vi "战舰胜利界面.vi"() -> ()   [LabVIEW 2018]
panel:
  out "失败界面":picture
  out "胜利界面":picture
  out "敌机是否入侵":bool
  out "得分":dbl
  out "战舰爆炸":picture
  out "血量":dbl
  out "战舰血量":T1 scale=0.0..100.0
  out "敌机爆炸":picture
  in  "敌机数量":dbl
  in  "敌机速度":dbl
  out "敌机":picture
  out "按键":dbl
  out "战舰":T2
  out "激光武器1":T3
  out "激光武器 2":T3
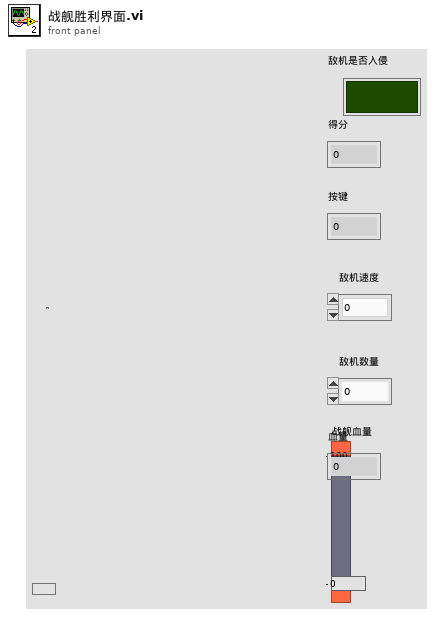
[diagram p1: front panel]
types:
  T1 = typedef "战列巡洋舰_血条.ctl" = dbl
  T2 = typedef "战列巡洋舰.ctl" = picture
  T3 = typedef "战列巡洋舰_激光武器.ctl" = picture
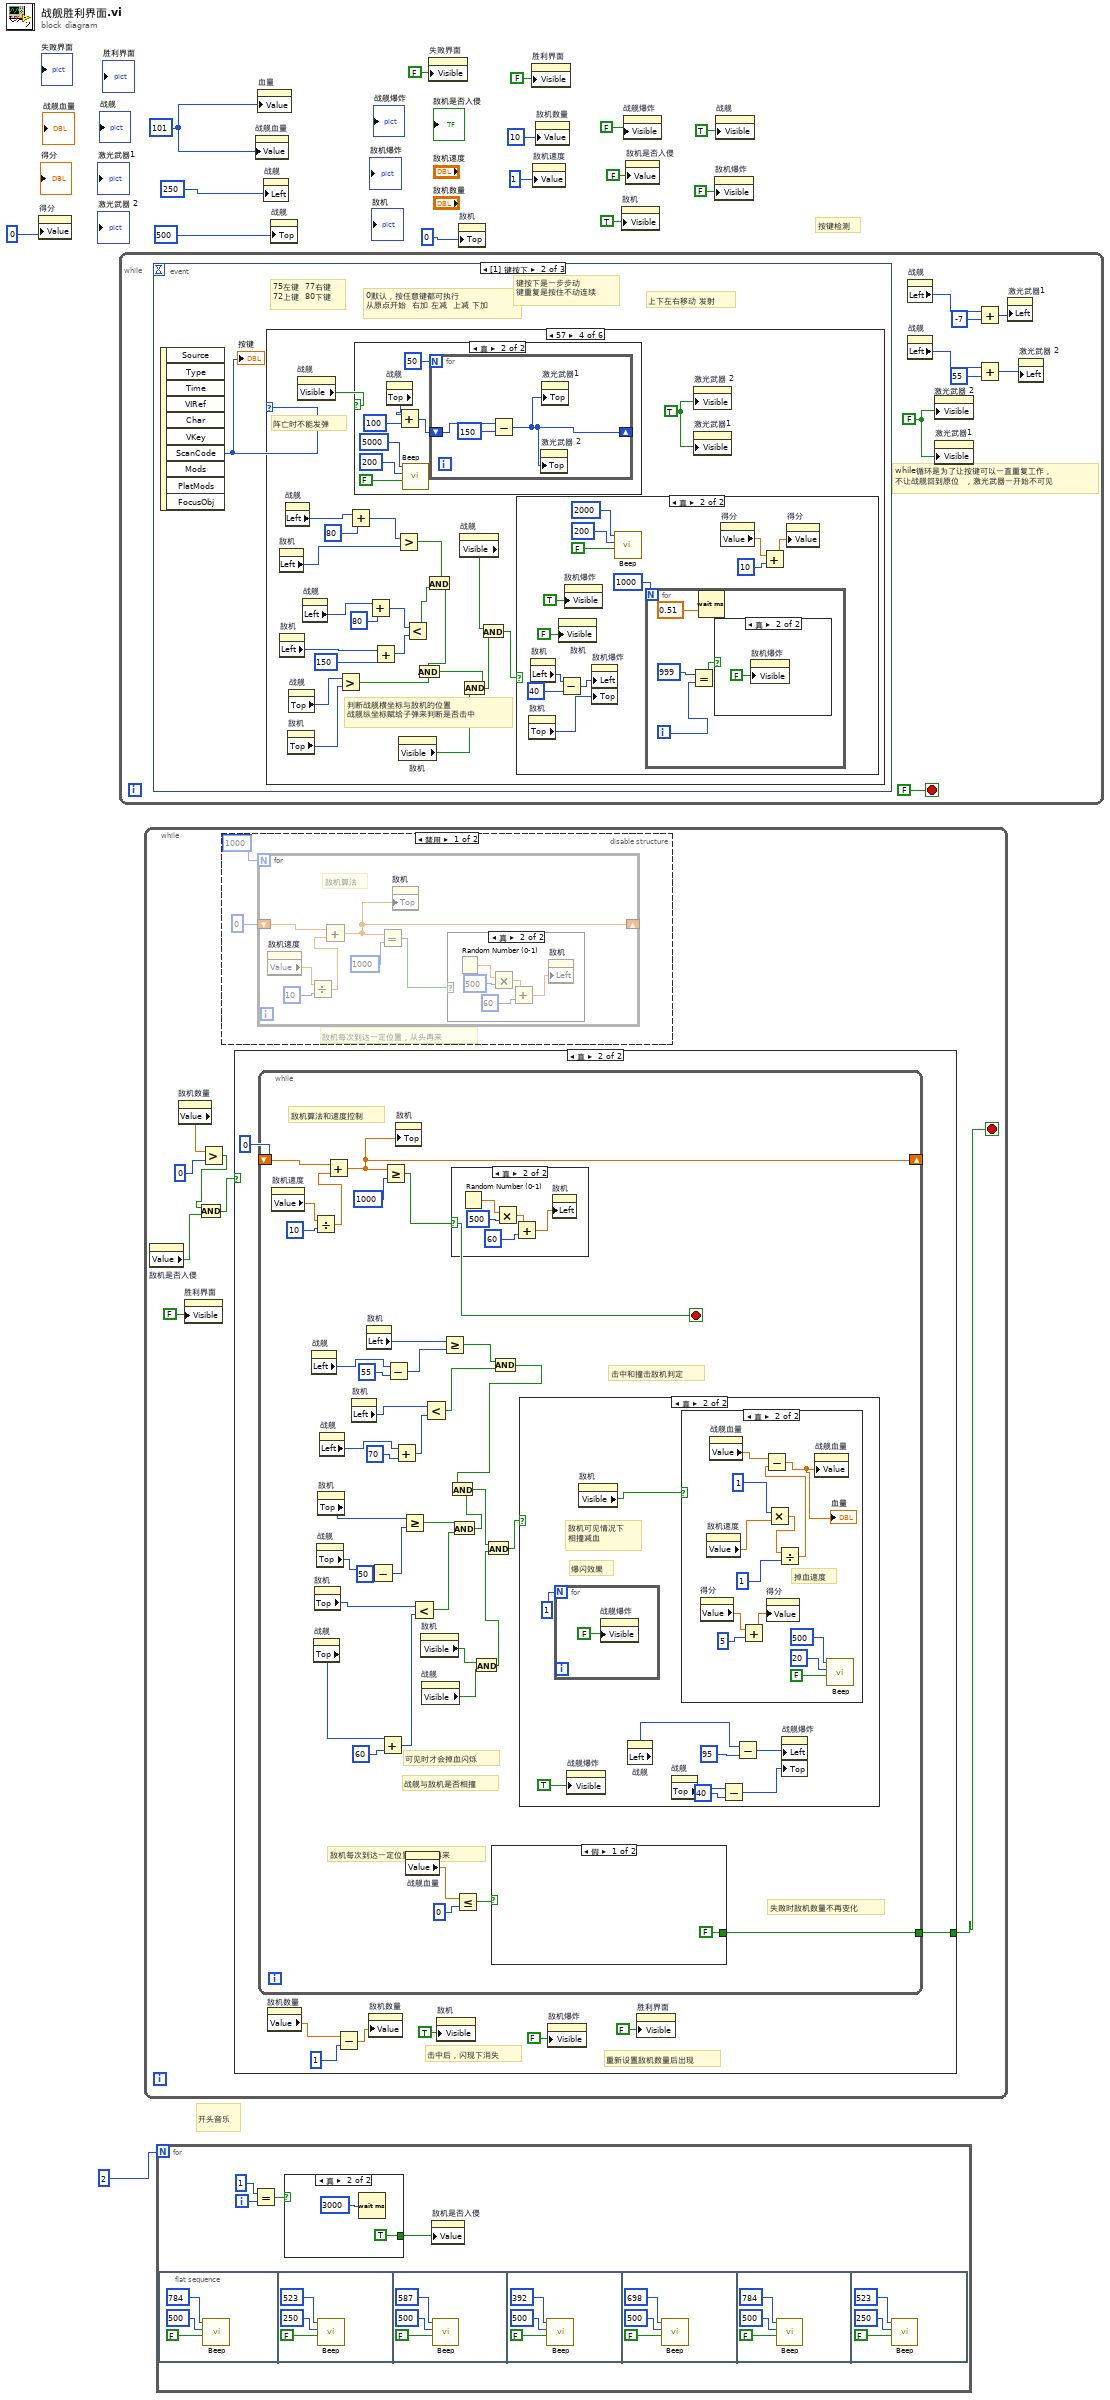
[diagram p0: block diagram]
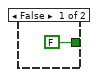
[diagram p2: hidden frame]
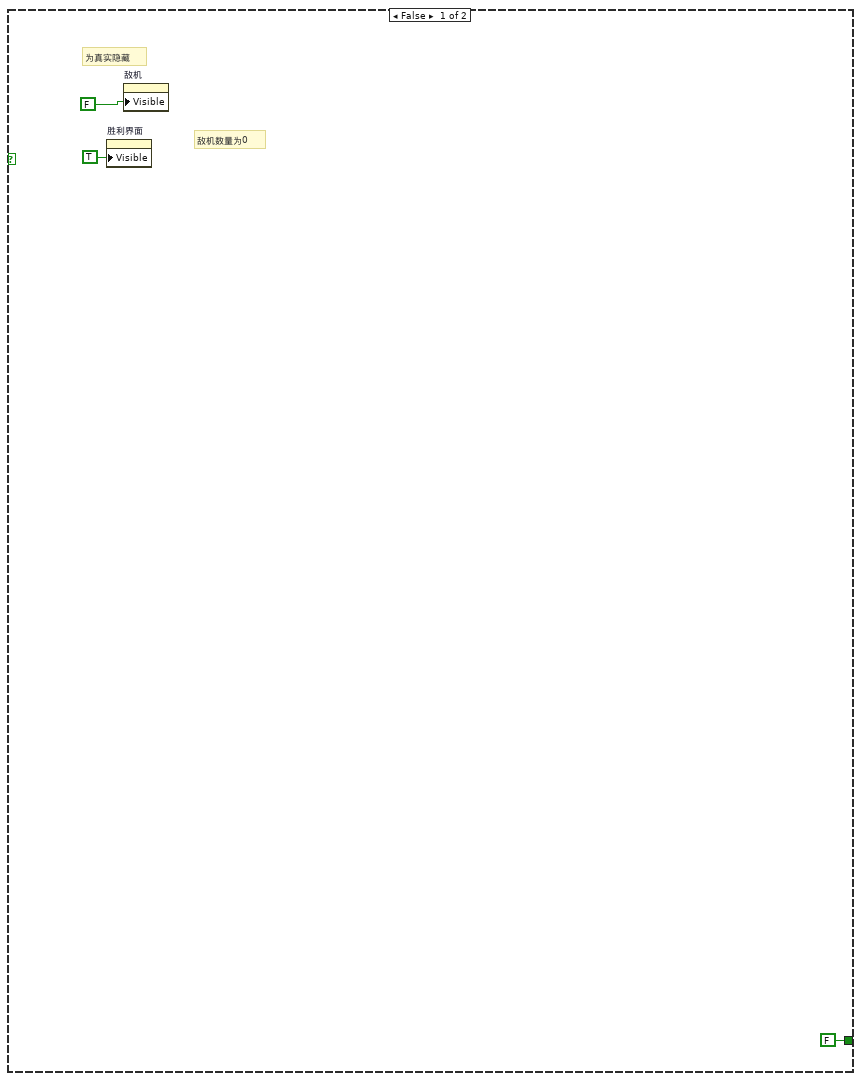
[diagram p3: hidden frame]
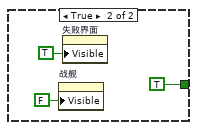
[diagram p4: hidden frame]
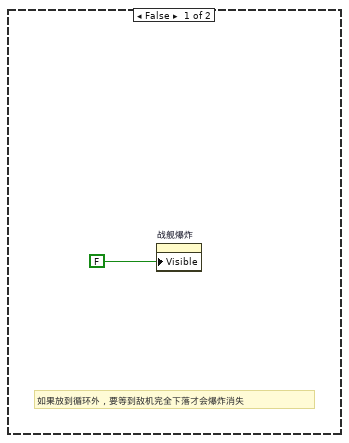
[diagram p5: hidden frame]
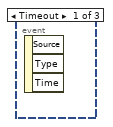
[diagram p10: hidden frame]
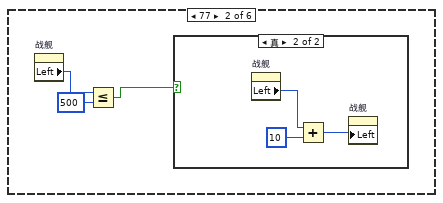
[diagram p12: hidden frame]
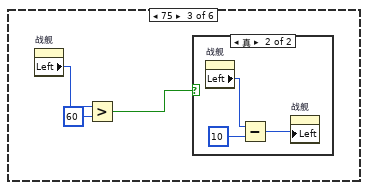
[diagram p14: hidden frame]
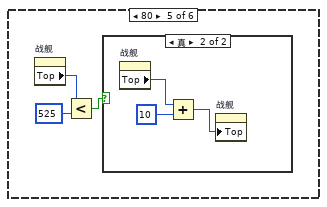
[diagram p19: hidden frame]
diagram:
  w9 = 101
  # "开头音乐"
  # "按键检测"
  n1 = property on="得分" class="DigNum (严格)"("Value"=0) -> ()  [unwired: 2 in, 2 out]
  n2 = while {
    stop <- FALSE stop-if-true
    w16 = FALSE
    # "while循环是为了让按键可以一直重复工作，\n不让战舰回到原位  ，激光武器一开始不可见"
    n3 = event shown="[1] 键按下" {
      selector: _ -> [_ _ _]
      dyn-events: _ -> [_ _ _]
      timeout: _ -> [_ _ _]
      event Timeout {
        n4 = event-data() -> ()  [unwired: 1 in, 3 out]
      }
      event Key Down {
        # "上下左右移动 发射"
        # "键按下是一步步动\n键重复是按住不动连续"
        # "75左键  77右键\n72上键  80下键"
        # "0默认，按任意键都可执行\n从原点开始  右加 左减  上减 下加"
        n5 = event-data() -> ("ScanCode"=w24:i16)  [unwired: 1 in, 9 out]
        "按键" <- w24
        n6 = case shown="57" w24 {
          frame 0, Default {
          }
          frame 77 {
            n7 = property on="战舰" class="Pict (严格)"() -> ("Left"=w27:i32)  [unwired: 2 in, 2 out]
            n8 = Less Or Equal?(x=w27, y=500) -> (x <= y?=w25:bool)
            n9 = case shown="真" w25 {
              frame False {
              }
              frame True {
                n10 = property on="战舰" class="Pict (严格)"() -> ("Left"=w29:i32)  [unwired: 2 in, 2 out]
                n11 = Add(x=w29, y=10) -> (x+y=w30:i32)
                n12 = property on="战舰" class="Pict (严格)"("Left"=w30) -> ()  [unwired: 2 in, 2 out]
              }
            }
          }
          frame 75 {
            n13 = property on="战舰" class="Pict (严格)"() -> ("Left"=w33:i32)  [unwired: 2 in, 2 out]
            n14 = Greater?(x=w33, y=60) -> (0:w31:bool)
            n15 = case shown="真" w31 {
              frame False {
              }
              frame True {
                n16 = property on="战舰" class="Pict (严格)"() -> ("Left"=w35:i32)  [unwired: 2 in, 2 out]
                n17 = Subtract(x=w35, y=10) -> (x-y=w36:i32)
                n18 = property on="战舰" class="Pict (严格)"("Left"=w36) -> ()  [unwired: 2 in, 2 out]
              }
            }
          }
          frame 57 {
            w59 = TRUE
            # "阵亡时不能发弹"
            # "判断战舰横坐标与敌机的位置\n战舰纵坐标赋给子弹来判断是否击中"
            n19 = property on="敌机" class="Pict"() -> ("Left"=w56:i32)  [unwired: 2 in, 2 out]
            n20 = property on="敌机" class="Pict"() -> ("Left"=w49:i32)  [unwired: 2 in, 2 out]
            n21 = property on="战舰" class="Pict (严格)"() -> ("Left"=w58:i32)  [unwired: 2 in, 2 out]
            n22 = property on="敌机" class="Pict"() -> ("Top"=w43:i32)  [unwired: 2 in, 2 out]
            n23 = property on="战舰" class="Pict (严格)"() -> ("Top"=w44:i32)  [unwired: 2 in, 2 out]
            n24 = property on="战舰" class="Pict (严格)"() -> ("Visible"=w37:bool)  [unwired: 2 in, 2 out]
            n25 = property on="战舰" class="Pict (严格)"() -> ("Left"=w51:i32)  [unwired: 2 in, 2 out]
            n26 = Greater?(x=w44, y=w43) -> (0:w45:bool)
            n27 = Add(x=w58, y=80) -> (x+y=w55:i32)
            n28 = case shown="真" w37 {
              frame False {
              }
              frame True {
                n29 = property on="战舰" class="Pict (严格)"() -> ("Top"=w65:i32)  [unwired: 2 in, 2 out]
                n30 = Add(x=w65, y=100) -> (x+y=w63:i32)
                n31 = call <vilib>:"Beep.vi"("use system alert? (T)"=FALSE, "duration (msec)"=u32 200, "frequency (Hz)"=u32 5000) -> ()  [unwired: 9 in]
                n32 = for {
                  N: 50 -> [_]
                  shift-right: [w67] -> _
                  shift-left: w63 -> [w69]
                  n33 = Subtract(x=w69, y=150) -> (x-y=w67:i32)
                  n34 = property on="激光武器 2" class="Pict (严格)"("Top"=w67) -> ()  [unwired: 2 in, 2 out]
                  n35 = property on="激光武器1" class="Pict (严格)"("Top"=w67) -> ()  [unwired: 2 in, 2 out]
                }
              }
            }
            n36 = Add(x=w51, y=80) -> (x+y=w53:i32)
            n37 = Add(x=w49, y=150) -> (x+y=w48:i32)
            n38 = Greater?(x=w55, y=w56) -> (0:w54:bool)
            n39 = property on="敌机" class="Pict"() -> ("Visible"=w41:bool)  [unwired: 2 in, 2 out]
            n40 = Less?(x=w53, y=w48) -> (x < y?=w50:bool)
            n41 = And(x=w54, y=w50) -> (x .and. y?=w46:bool)
            n42 = And(x=w46, y=w45) -> (x .and. y?=w42:bool)
            n43 = property on="战舰" class="Pict (严格)"() -> ("Visible"=w40:bool)  [unwired: 2 in, 2 out]
            n44 = And(x=w42, y=w41) -> (x .and. y?=w39:bool)
            n45 = And(x=w40, y=w39) -> (x .and. y?=w38:bool)
            n46 = case shown="真" w38 {
              frame False {
              }
              frame True {
                n47 = property on="敌机" class="Pict"() -> ("Top"=w80:i32)  [unwired: 2 in, 2 out]
                n48 = property on="敌机" class="Pict"() -> ("Left"=w78:i32)  [unwired: 2 in, 2 out]
                n49 = property on="敌机" class="Pict"("Visible"=FALSE ("可见")) -> ()  [unwired: 2 in, 2 out]
                n50 = Subtract(x=w78, y=40) -> (x-y=w77:i32)
                n51 = property on="敌机爆炸" class="Pict"("Visible"=TRUE ("可见")) -> ()  [unwired: 2 in, 2 out]
                n52 = property on="敌机爆炸" class="Pict"("Left"=w77, "Top"=w80) -> ()  [unwired: 2 in, 2 out]
                n53 = call <vilib>:"Beep.vi"("use system alert? (T)"=FALSE, "duration (msec)"=u32 200, "frequency (Hz)"=u32 2000) -> ()  [unwired: 9 in]
                n54 = for {
                  N: 1000 -> [_]
                  i -> [w85]
                  n55 = Equal?(x=999, y=w85) -> (x = y?=w86:bool)
                  n56 = Wait (ms)(milliseconds to wait=0.51) -> ()  [unwired: 1 out]
                  n57 = case shown="真" w86 {
                    frame False {
                    }
                    frame True {
                      n58 = property on="敌机爆炸" class="Pict"("Visible"=FALSE ("可见")) -> ()  [unwired: 2 in, 2 out]
                    }
                  }
                }
                n59 = property on="得分" class="DigNum (严格)"() -> ("Value"=w75:dbl)  [unwired: 2 in, 2 out]
                n60 = Add(x=w75, y=10) -> (x+y=w73:dbl)
                n61 = property on="得分" class="DigNum (严格)"("Value"=w73) -> ()  [unwired: 2 in, 2 out]
              }
            }
            n62 = property on="激光武器 2" class="Pict (严格)"("Visible"=w59) -> ()  [unwired: 2 in, 2 out]
            n63 = property on="激光武器1" class="Pict (严格)"("Visible"=w59) -> ()  [unwired: 2 in, 2 out]
          }
          frame 80 {
            n64 = property on="战舰" class="Pict (严格)"() -> ("Top"=w90:i32)  [unwired: 2 in, 2 out]
            n65 = Less?(x=w90, y=525) -> (x < y?=w88:bool)
            n66 = case shown="真" w88 {
              frame False {
              }
              frame True {
                n67 = property on="战舰" class="Pict (严格)"() -> ("Top"=w92:i32)  [unwired: 2 in, 2 out]
                n68 = Add(x=w92, y=10) -> (x+y=w91:i32)
                n69 = property on="战舰" class="Pict (严格)"("Top"=w91) -> ()  [unwired: 2 in, 2 out]
              }
            }
          }
          frame 72 {
            n70 = property on="战舰" class="Pict (严格)"() -> ("Top"=w96:i32)  [unwired: 2 in, 2 out]
            n71 = Greater Or Equal?(x=w96, y=25) -> (x >= y?=w95:bool)
            n72 = case shown="真" w95 {
              frame False {
              }
              frame True {
                n73 = property on="战舰" class="Pict (严格)"() -> ("Top"=w99:i32)  [unwired: 2 in, 2 out]
                n74 = Subtract(x=w99, y=10) -> (x-y=w98:i32)
                n75 = property on="战舰" class="Pict (严格)"("Top"=w98) -> ()  [unwired: 2 in, 2 out]
              }
            }
          }
        }
      }
      event Key Repeat {
        # "75左键  77右键\n72上键  80下键\n空格 57"
        # "0默认，按任意键都可执行\n从原点开始  右加 左减  上减 下加"
        n76 = event-data() -> ("ScanCode"=w100:i16)  [unwired: 1 in, 9 out]
        n77 = case shown="72" w100 {
          frame 0, Default {
          }
          frame 77 {
            n78 = property on="战舰" class="Pict (严格)"() -> ("Left"=w103:i32)  [unwired: 2 in, 2 out]
            n79 = Less Or Equal?(x=w103, y=500) -> (x <= y?=w102:bool)
            n80 = case shown="真" w102 {
              frame False {
              }
              frame True {
                n81 = property on="战舰" class="Pict (严格)"() -> ("Left"=w105:i32)  [unwired: 2 in, 2 out]
                n82 = Add(x=w105, y=10) -> (x+y=w106:i32)
                n83 = property on="战舰" class="Pict (严格)"("Left"=w106) -> ()  [unwired: 2 in, 2 out]
              }
            }
          }
          frame 75 {
            n84 = property on="战舰" class="Pict (严格)"() -> ("Left"=w109:i32)  [unwired: 2 in, 2 out]
            n85 = Greater Or Equal?(x=w109, y=25) -> (x >= y?=w108:bool)
            n86 = case shown="真" w108 {
              frame False {
              }
              frame True {
                n87 = property on="战舰" class="Pict (严格)"() -> ("Left"=w112:i32)  [unwired: 2 in, 2 out]
                n88 = Subtract(x=w112, y=10) -> (x-y=w111:i32)
                n89 = property on="战舰" class="Pict (严格)"("Left"=w111) -> ()  [unwired: 2 in, 2 out]
              }
            }
          }
          frame 80 {
            n90 = property on="战舰" class="Pict (严格)"() -> ("Top"=w115:i32)  [unwired: 2 in, 2 out]
            n91 = Less Or Equal?(x=w115, y=525) -> (x <= y?=w114:bool)
            n92 = case shown="真" w114 {
              frame False {
              }
              frame True {
                n93 = property on="战舰" class="Pict (严格)"() -> ("Top"=w117:i32)  [unwired: 2 in, 2 out]
                n94 = Add(x=w117, y=10) -> (x+y=w116:i32)
                n95 = property on="战舰" class="Pict (严格)"("Top"=w116) -> ()  [unwired: 2 in, 2 out]
              }
            }
          }
          frame 72 {
            n96 = property on="战舰" class="Pict (严格)"() -> ("Top"=w121:i32)  [unwired: 2 in, 2 out]
            n97 = Greater Or Equal?(x=w121, y=25) -> (x >= y?=w120:bool)
            n98 = case shown="真" w120 {
              frame False {
              }
              frame True {
                n99 = property on="战舰" class="Pict (严格)"() -> ("Top"=w124:i32)  [unwired: 2 in, 2 out]
                n100 = Subtract(x=w124, y=10) -> (x-y=w123:i32)
                n101 = property on="战舰" class="Pict (严格)"("Top"=w123) -> ()  [unwired: 2 in, 2 out]
              }
            }
          }
        }
      }
    }
    n102 = property on="战舰" class="Pict (严格)"() -> ("Left"=w22:i32)  [unwired: 2 in, 2 out]
    n103 = property on="战舰" class="Pict (严格)"() -> ("Left"=w18:i32)  [unwired: 2 in, 2 out]
    n104 = property on="激光武器 2" class="Pict (严格)"("Visible"=w16) -> ()  [unwired: 2 in, 2 out]
    n105 = property on="激光武器1" class="Pict (严格)"("Visible"=w16) -> ()  [unwired: 2 in, 2 out]
    n106 = Add(x=w22, y=-7) -> (x+y=w21:i32)
    n107 = Add(x=w18, y=55) -> (x+y=w17:i32)
    n108 = property on="激光武器1" class="Pict (严格)"("Left"=w21) -> ()  [unwired: 2 in, 2 out]
    n109 = property on="激光武器 2" class="Pict (严格)"("Left"=w17) -> ()  [unwired: 2 in, 2 out]
  }
  n110 = while {
    stop <- w126 stop-if-true
    n111 = property on="敌机是否入侵" class="Bool (严格)"() -> ("Value"=w129:bool)  [unwired: 2 in, 2 out]
    n112 = property on="敌机数量" class="DigNum (严格)"() -> ("Value"=w131:dbl)  [unwired: 2 in, 2 out]
    n113 = property on="胜利界面" class="Pict"("Visible"=FALSE ("可见")) -> ()  [unwired: 2 in, 2 out]
    n114 = Greater?(x=w131, y=0) -> (0:w128:bool)
    n115 = And(x=w128, y=w129) -> (x .and. y?=w127:bool)
    n116 = disable-structure shown="禁用" {
      frame Disabled {
        # "敌机每次到达一定位置，从头再来"
        n117 = for {
          N: 1000 -> [_]
          shift-right: [w219] -> _
          shift-left: 0 -> [w222]
          # "敌机算法"
          n118 = property on="敌机速度" class="DigNum (严格)"() -> ("Value"=w218:dbl)  [unwired: 2 in, 2 out]
          n119 = Divide(x=w218, y=10) -> (x/y=w217:dbl)
          n120 = Add(x=w222, y=w217) -> (x+y=w219:dbl)
          n121 = Equal?(x=w219, y=1000) -> (x = y?=w220:bool)
          n122 = property on="敌机" class="Pict"("Top"=w219) -> ()  [unwired: 2 in, 2 out]
          n123 = case shown="真" w220 {
            frame False {
            }
            frame True {
              n124 = Random Number (0-1)() -> (number: 0 to 1=w227:dbl)
              n125 = Multiply(x=w227, y=500) -> (x*y=w225:dbl)
              n126 = Add(x=w225, y=60) -> (x+y=w224:dbl)
              n127 = property on="敌机" class="Pict"("Left"=w224) -> ()  [unwired: 2 in, 2 out]
            }
          }
        }
      }
      frame Enabled {
      }
    }
    n128 = case shown="真" w127 {
      tunnel: [FALSE w135] -> w126
      frame False {
        # "敌机数量为0"
        # "为真实隐藏"
        n129 = property on="胜利界面" class="Pict"("Visible"=TRUE ("可见")) -> ()  [unwired: 2 in, 2 out]
        n130 = property on="敌机" class="Pict"("Visible"=FALSE ("可见")) -> ()  [unwired: 2 in, 2 out]
      }
      frame True {
        # "重新设置敌机数量后出现"
        # "击中后，闪现下消失"
        # "敌机每次到达一定位置，从头再来"
        n131 = while {
          shift-right: [w178] -> _
          shift-left: 0 -> [w180]
          tunnel: [w143] -> w135
          stop <- w174 stop-if-true
          # "失败时敌机数量不再变化"
          # "击中和撞击敌机判定"
          # "可见时才会掉血闪烁"
          # "战舰与敌机是否相撞"
          # "敌机算法和速度控制"
          n132 = property on="敌机速度" class="DigNum (严格)"() -> ("Value"=w177:dbl)  [unwired: 2 in, 2 out]
          n133 = property on="战舰" class="Pict (严格)"() -> ("Left"=w172:i32)  [unwired: 2 in, 2 out]
          n134 = Divide(x=w177, y=10) -> (x/y=w176:dbl)
          n135 = property on="战舰" class="Pict (严格)"() -> ("Top"=w156:i32)  [unwired: 2 in, 2 out]
          n136 = property on="敌机" class="Pict"() -> ("Top"=w155:i32)  [unwired: 2 in, 2 out]
          n137 = property on="战舰" class="Pict (严格)"() -> ("Top"=w162:i32)  [unwired: 2 in, 2 out]
          n138 = property on="敌机" class="Pict"() -> ("Top"=w163:i32)  [unwired: 2 in, 2 out]
          n139 = property on="战舰" class="Pict (严格)"() -> ("Left"=w166:i32)  [unwired: 2 in, 2 out]
          n140 = Add(x=w180, y=w176) -> (x+y=w178:dbl)
          n141 = property on="敌机" class="Pict"() -> ("Left"=w168:i32)  [unwired: 2 in, 2 out]
          n142 = property on="敌机" class="Pict"() -> ("Left"=w173:i32)  [unwired: 2 in, 2 out]
          n143 = Subtract(x=w162, y=50) -> (x-y=w160:i32)
          n144 = Add(x=w156, y=60) -> (x+y=w158:i32)
          n145 = Greater Or Equal?(x=w178, y=1000) -> (x >= y?=w174:bool)
          n146 = Subtract(x=w172, y=55) -> (x-y=w171:i32)
          n147 = Add(x=w166, y=70) -> (x+y=w165:i32)
          n148 = property on="敌机" class="Pict"("Top"=w178) -> ()  [unwired: 2 in, 2 out]
          n149 = Greater Or Equal?(x=w163, y=w160) -> (x >= y?=w154:bool)
          n150 = property on="战舰血量" class="Slide (严格)"() -> ("Value"=w148:T1)  [unwired: 2 in, 2 out]
          n151 = Less?(x=w155, y=w158) -> (x < y?=w153:bool)
          n152 = property on="敌机" class="Pict"() -> ("Visible"=w146:bool)  [unwired: 2 in, 2 out]
          n153 = property on="战舰" class="Pict (严格)"() -> ("Visible"=w145:bool)  [unwired: 2 in, 2 out]
          n154 = Less?(x=w168, y=w165) -> (x < y?=w164:bool)
          n155 = Greater Or Equal?(x=w173, y=w171) -> (x >= y?=w169:bool)
          n156 = case shown="真" w174 {
            frame False {
            }
            frame True {
              n157 = Random Number (0-1)() -> (number: 0 to 1=w213:dbl)
              n158 = Multiply(x=w213, y=500) -> (x*y=w211:dbl)
              n159 = Add(x=w211, y=60) -> (x+y=w210:dbl)
              n160 = property on="敌机" class="Pict"("Left"=w210) -> ()  [unwired: 2 in, 2 out]
            }
          }
          n161 = And(x=w154, y=w153) -> (x .and. y?=w152:bool)
          n162 = Less Or Equal?(x=w148, y=0) -> (x <= y?=w149:bool)
          n163 = And(x=w146, y=w145) -> (x .and. y?=w144:bool)
          n164 = case shown="假" w149 {
            tunnel: [FALSE TRUE] -> w143
            frame False {
            }
            frame True {
              n165 = property on="战舰" class="Pict (严格)"("Visible"=FALSE ("可见")) -> ()  [unwired: 2 in, 2 out]
              n166 = property on="失败界面" class="Pict"("Visible"=TRUE ("可见")) -> ()  [unwired: 2 in, 2 out]
            }
          }
          n167 = And(x=w169, y=w164) -> (x .and. y?=w159:bool)
          n168 = And(x=w159, y=w152) -> (x .and. y?=w151:bool)
          n169 = And(x=w151, y=w144) -> (x .and. y?=w150:bool)
          n170 = case shown="真" w150 {
            frame False {
              # "如果放到循环外，要等到敌机完全下落才会爆炸消失"
              n171 = property on="战舰爆炸" class="Pict"("Visible"=FALSE ("可见")) -> ()  [unwired: 2 in, 2 out]
            }
            frame True {
              # "爆闪效果"
              # "敌机可见情况下\n相撞减血"
              n172 = for {
                N: 1 -> [_]
                n173 = property on="战舰爆炸" class="Pict"("Visible"=FALSE ("可见")) -> ()  [unwired: 2 in, 2 out]
              }
              n174 = property on="战舰爆炸" class="Pict"("Visible"=TRUE ("可见")) -> ()  [unwired: 2 in, 2 out]
              n175 = property on="敌机" class="Pict"() -> ("Visible"=w194:bool)  [unwired: 2 in, 2 out]
              n176 = property on="战舰" class="Pict (严格)"() -> ("Left"=w192:i32)  [unwired: 2 in, 2 out]
              n177 = property on="战舰" class="Pict (严格)"() -> ("Top"=w189:i32)  [unwired: 2 in, 2 out]
              n178 = case shown="真" w194 {
                frame False {
                }
                frame True {
                  # "掉血速度"
                  n179 = property on="得分" class="DigNum (严格)"() -> ("Value"=w201:dbl)  [unwired: 2 in, 2 out]
                  n180 = property on="敌机速度" class="DigNum (严格)"() -> ("Value"=w207:dbl)  [unwired: 2 in, 2 out]
                  n181 = property on="战舰血量" class="Slide (严格)"() -> ("Value"=w208:T1)  [unwired: 2 in, 2 out]
                  n182 = Add(x=w201, y=5) -> (x+y=w200:dbl)
                  n183 = Multiply(x=1, y=w207) -> (x*y=w206:dbl)
                  n184 = property on="得分" class="DigNum (严格)"("Value"=w200) -> ()  [unwired: 2 in, 2 out]
                  n185 = Divide(x=w206, y=1) -> (x/y=w203:dbl)
                  n186 = Subtract(x=w208, y=w203) -> (x-y=w202:T1)
                  "血量" <- w202
                  n187 = property on="战舰血量" class="Slide (严格)"("Value"=w202) -> ()  [unwired: 2 in, 2 out]
                  n188 = call <vilib>:"Beep.vi"("use system alert? (T)"=FALSE, "duration (msec)"=u32 20, "frequency (Hz)"=u32 500) -> ()  [unwired: 9 in]
                }
              }
              n189 = Subtract(x=w189, y=40) -> (x-y=w187:i32)
              n190 = Subtract(x=w192, y=95) -> (x-y=w190:i32)
              n191 = property on="战舰爆炸" class="Pict"("Left"=w190, "Top"=w187) -> ()  [unwired: 2 in, 2 out]
            }
          }
        }
        n192 = property on="敌机数量" class="DigNum (严格)"() -> ("Value"=w140:dbl)  [unwired: 2 in, 2 out]
        n193 = Subtract(x=w140, y=1) -> (x-y=w141:dbl)
        n194 = property on="敌机数量" class="DigNum (严格)"("Value"=w141) -> ()  [unwired: 2 in, 2 out]
        n195 = property on="敌机" class="Pict"("Visible"=TRUE ("可见")) -> ()  [unwired: 2 in, 2 out]
        n196 = property on="敌机爆炸" class="Pict"("Visible"=FALSE ("可见")) -> ()  [unwired: 2 in, 2 out]
        n197 = property on="胜利界面" class="Pict"("Visible"=FALSE ("可见")) -> ()  [unwired: 2 in, 2 out]
      }
    }
  }
  n198 = for {
    N: 2 -> [_]
    i -> [w229]
    n199 = flat-sequence {
      frame #0 {
        n200 = call <vilib>:"Beep.vi"("use system alert? (T)"=FALSE, "duration (msec)"=500, "frequency (Hz)"=784) -> ()  [unwired: 9 in]
      }
      frame #1 {
        n201 = call <vilib>:"Beep.vi"("use system alert? (T)"=FALSE, "duration (msec)"=250, "frequency (Hz)"=523) -> ()  [unwired: 9 in]
      }
      frame #2 {
        n202 = call <vilib>:"Beep.vi"("use system alert? (T)"=FALSE, "duration (msec)"=500, "frequency (Hz)"=587) -> ()  [unwired: 9 in]
      }
      frame #3 {
        n203 = call <vilib>:"Beep.vi"("use system alert? (T)"=FALSE, "duration (msec)"=500, "frequency (Hz)"=392) -> ()  [unwired: 9 in]
      }
      frame #4 {
        n204 = call <vilib>:"Beep.vi"("use system alert? (T)"=FALSE, "duration (msec)"=500, "frequency (Hz)"=698) -> ()  [unwired: 9 in]
      }
      frame #5 {
        n205 = call <vilib>:"Beep.vi"("use system alert? (T)"=FALSE, "duration (msec)"=500, "frequency (Hz)"=784) -> ()  [unwired: 9 in]
      }
      frame #6 {
        n206 = call <vilib>:"Beep.vi"("use system alert? (T)"=FALSE, "duration (msec)"=250, "frequency (Hz)"=523) -> ()  [unwired: 9 in]
      }
    }
    n207 = Equal?(x=1, y=w229) -> (x = y?=w231:bool)
    n208 = case shown="真" w231 {
      tunnel: [FALSE ("敌机是否入侵") TRUE ("敌机是否入侵")] -> w228
      frame False {
      }
      frame True {
        n209 = Wait (ms)(milliseconds to wait=u32 3000 ("等待时间（毫秒）")) -> ()  [unwired: 1 out]
      }
    }
    n210 = property on="敌机是否入侵" class="Bool (严格)"("Value"=w228) -> ()  [unwired: 2 in, 2 out]
  }
  n211 = property on="战舰血量" class="Slide (严格)"("Value"=w9) -> ()  [unwired: 2 in, 2 out]
  n212 = property on="血量" class="DigNum (严格)"("Value"=w9) -> ()  [unwired: 2 in, 2 out]
  n213 = property on="战舰" class="Pict (严格)"("Left"=250 ("位置:居左")) -> ()  [unwired: 2 in, 2 out]
  n214 = property on="战舰" class="Pict (严格)"("Top"=500 ("位置:置顶")) -> ()  [unwired: 2 in, 2 out]
  n215 = property on="失败界面" class="Pict"("Visible"=FALSE ("可见")) -> ()  [unwired: 2 in, 2 out]
  n216 = property on="敌机" class="Pict"("Top"=0) -> ()  [unwired: 2 in, 2 out]
  n217 = property on="胜利界面" class="Pict"("Visible"=FALSE ("可见")) -> ()  [unwired: 2 in, 2 out]
  n218 = property on="敌机速度" class="DigNum (严格)"("Value"=1) -> ()  [unwired: 2 in, 2 out]
  n219 = property on="敌机数量" class="DigNum (严格)"("Value"=10) -> ()  [unwired: 2 in, 2 out]
  n220 = property on="敌机" class="Pict"("Visible"=TRUE ("可见")) -> ()  [unwired: 2 in, 2 out]
  n221 = property on="战舰爆炸" class="Pict"("Visible"=FALSE ("可见")) -> ()  [unwired: 2 in, 2 out]
  n222 = property on="敌机是否入侵" class="Bool (严格)"("Value"=FALSE ("敌机是否入侵")) -> ()  [unwired: 2 in, 2 out]
  n223 = property on="敌机爆炸" class="Pict"("Visible"=FALSE ("可见")) -> ()  [unwired: 2 in, 2 out]
  n224 = property on="战舰" class="Pict (严格)"("Visible"=TRUE ("可见")) -> ()  [unwired: 2 in, 2 out]
